vi "find all matching strings in the list.vi"(10 "regular expression":string="^.*?bg.*", 11 "strings":string[](array[string])=["aaa", "bgf", "ert", "vvbg", "nhtn", "yuk"]) -> (1 "at least one match found":bool=TRUE, 2 "list of matching string index":i32[](array[numeric])=[1, 3], 3 "list of matching strings":string[](array[string])=["bgf", "vvbg"])   [LabVIEW 2015]
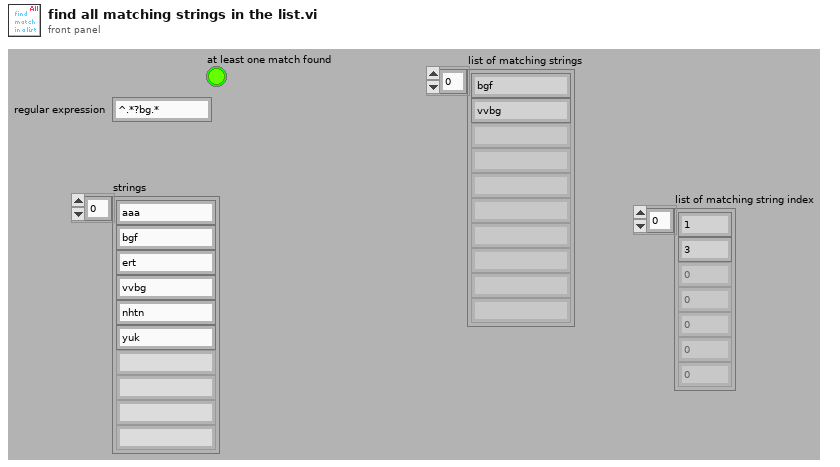
[diagram p1: front panel]
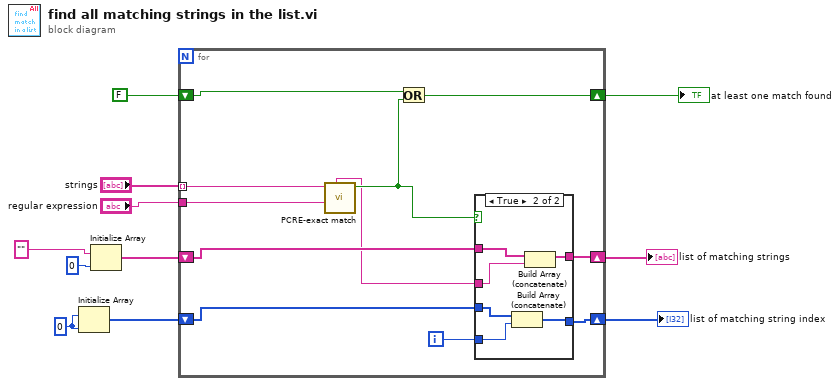
[diagram p0: block diagram]
diagram:
  w5 = 0 ("dimension size")
  n1 = Initialize Array(w5, w5) -> (w4:i32[])
  n2 = Initialize Array("" ("regular expression"), 0 ("dimension size")) -> (w8:string[])
  n3 = for {
    tunnel: "strings" -> [w22] mode=indexing
    tunnel: "regular expression" -> [w21]
    shift-right: [w17] -> w2
    shift-left: w8 -> [w16]
    shift-right: [w20] -> w10
    shift-left: FALSE -> [w19]
    shift-right: [w15] -> w3
    shift-left: w4 -> [w14]
    i -> [w13]
    n4 = call "PCRE-exact match.vi"("regular expression"=w21, "input string"=w22) -> ("exact match"=w18:bool, "output string"=w12:string)  [unwired: 7 in, 1 out]
    n5 = Or(x=w19, y=w18) -> (x .or. y?=w20:bool)
    n6 = case shown="True" w18 {
      tunnel: [w24 w25] -> w17
      tunnel: w16 -> [w24 w27]
      tunnel: [w23 w29] -> w15
      tunnel: w14 -> [w23 w30]
      tunnel: w13 -> [_ w28]
      tunnel: w12 -> [_ w26]
      frame False {
      }
      frame True {
        n7 = Build Array (concatenate)(w30, w28) -> (w29:i32[])
        n8 = Build Array (concatenate)(w27, w26) -> (w25:string[])
      }
    }
  }
  "at least one match found" <- w10
  "list of matching string index" <- w3
  "list of matching strings" <- w2
